vi "excelFile_Create.vi"(8 "error in (no error)":errorcluster, 9 "fileType":T1, 10 "Path":path, 11 "reference in":refnum<class "excelFile.lvclass">) -> (0 "error out":errorcluster, 3 "reference out":refnum<class "excelFile.lvclass">)   [LabVIEW 2015, in "excelFile.lvclass"]
doc: "Constructor."
uses:
  excelFile.lvclass
  fileType.ctl
  <vilib>/addons/_AddQ/G#Object/utils/G#Object_CreateMethod.ctl
  <vilib>/addons/_AddQ/G#Object/G#Object.lvclass
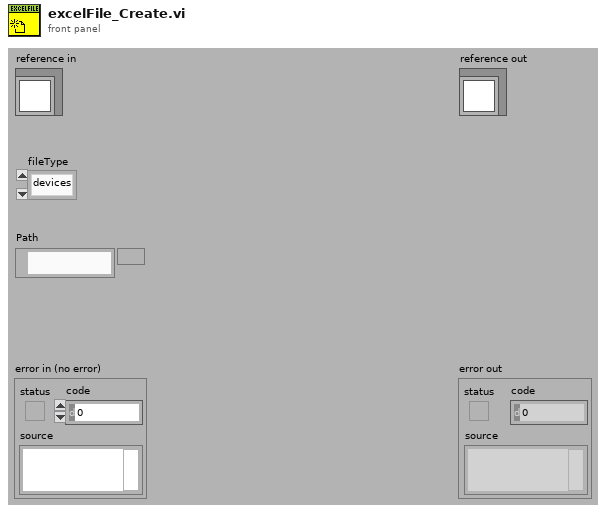
[diagram p1: front panel]
types:
  T1 = typedef "excelFile.lvclass/fileType.ctl" = enum16{"devices", "items", "partsTracking", "TSR"}
  T2 = typedef "G#Object.lvclass/G#Object_CreateMethod.ctl" = enum16{"Create", "Create or look up existing", "Look up existing"}
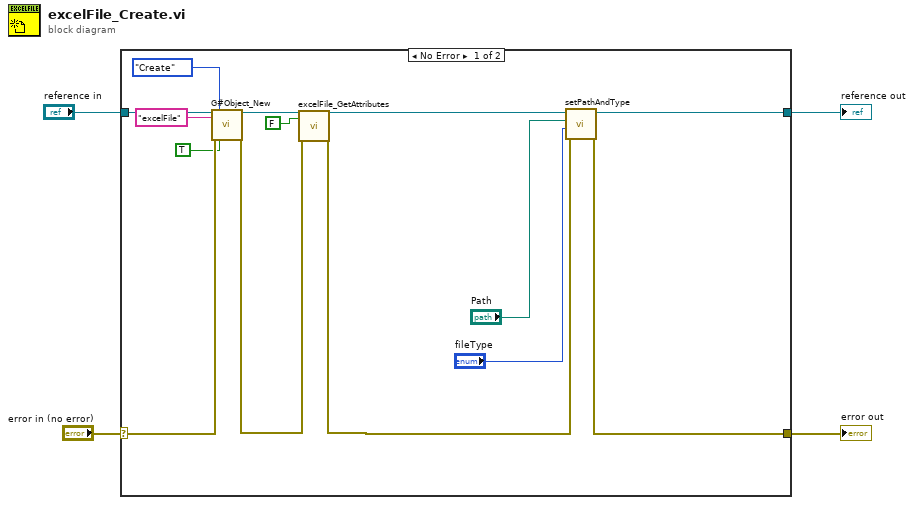
[diagram p0: block diagram]
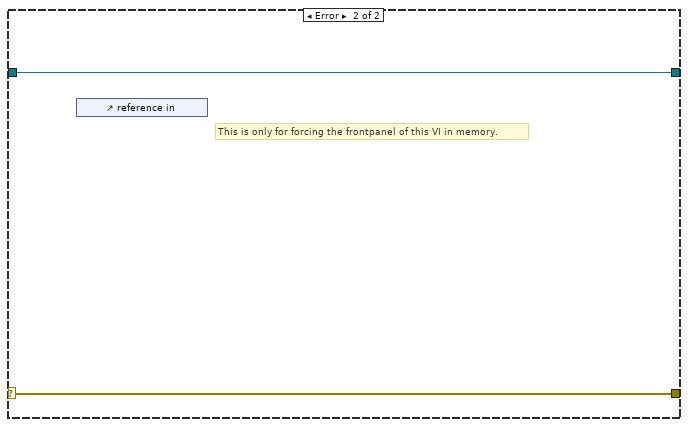
[diagram p2: hidden frame]
diagram:
  n1 = case shown="No Error" "error in (no error)" {
    selector: "error in (no error)" -> [w17 w20]
    tunnel: [w12 w20] -> w3
    tunnel: [w5 w19] -> w1
    tunnel: "reference in" -> [w18 w19]
    frame No Error {
      n2 = call <vilib>:"G#Object_New.vi"("reference in"=w18, "object name"="excelFile", "error in (no error)"=w17, "create method"=G#Object_CreateMethod."Create", "user counter (T)?"=TRUE ("User Counter")) -> ("reference out"=w15:refnum<class "excelFile.lvclass">, "error out"=w14:errorcluster)  [unwired: 12 in, 1 out]
      n3 = call "excelFile_GetAttributes.vi"("reference in"=w15, "return data? (T)"=FALSE ("return data"), "error in (no error)"=w14) -> ("reference out"=w10:refnum<class "excelFile.lvclass">, "error out"=w7:errorcluster)  [unwired: 13 in, 2 out]
      n4 = call "setPathAndType.vi"("error in (no error)"=w7, "fileType"="fileType", "Path"="Path", "reference in"=w10) -> ("error out"=w12:errorcluster, "reference out"=w5:refnum<class "excelFile.lvclass">)  [unwired: 6 in]
    }
    frame Error {
      # "This is only for forcing the frontpanel of this VI in memory."
      n5 = control-ref of="reference in"() -> ()  [unwired: 1 out]
    }
  }
  "error out" <- w3
  "reference out" <- w1
